vi "Go to Setpoint.vi"() -> ()   [LabVIEW 2010]
panel:
  out "error out":errorcluster
  in  "error in (no error)":errorcluster
  in  "Air Temperature Setpoint (°C)":dbl=37.5 min=25.0 max=80.0 step=0.1
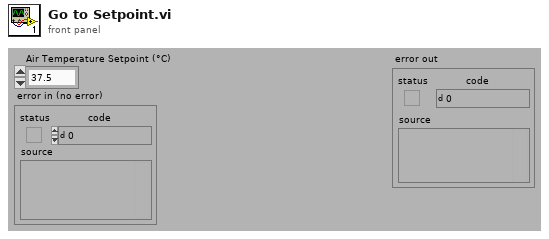
[diagram p1: front panel]
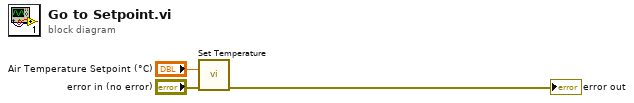
[diagram p0: block diagram]
diagram:
  n1 = call "Set Temperature.vi"("Air Temperature Setpoint (°C)"="Air Temperature Setpoint (°C)", "error in (no error)"="error in (no error)") -> ("error out"=→"error out":errorcluster)  [unwired: 13 in]
